vi "Time String to Millisecond.vi"(8 "Error in":errorcluster caption="Error in (no error)", 11 "Parameter":string="1min 30s 20ms") -> (0 "Error out":errorcluster, 2 "Array":string[](array[string]), 3 "sum":i64)   [LabVIEW 2020, in "CSMStand(Lite).lvlib"]
uses:
  CSMStand(Lite).lvlib
  <userlib>/_NEVSTOP/Communicable State Machine(CSM)/addons/API-String-Arugments-Support/API String Arguments Support.lvlib
  <userlib>/_NEVSTOP/Communicable State Machine(CSM)/_Shared/CSM Shared.lvlib
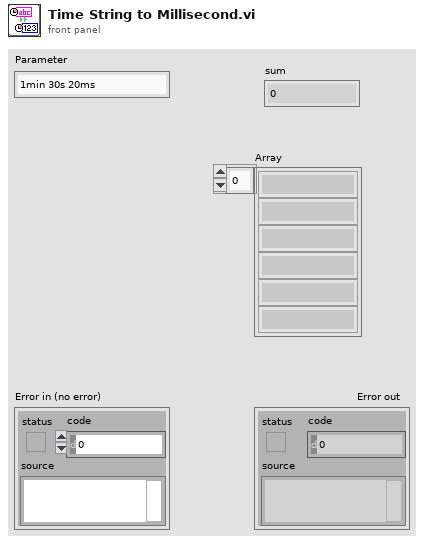
[diagram p1: front panel]
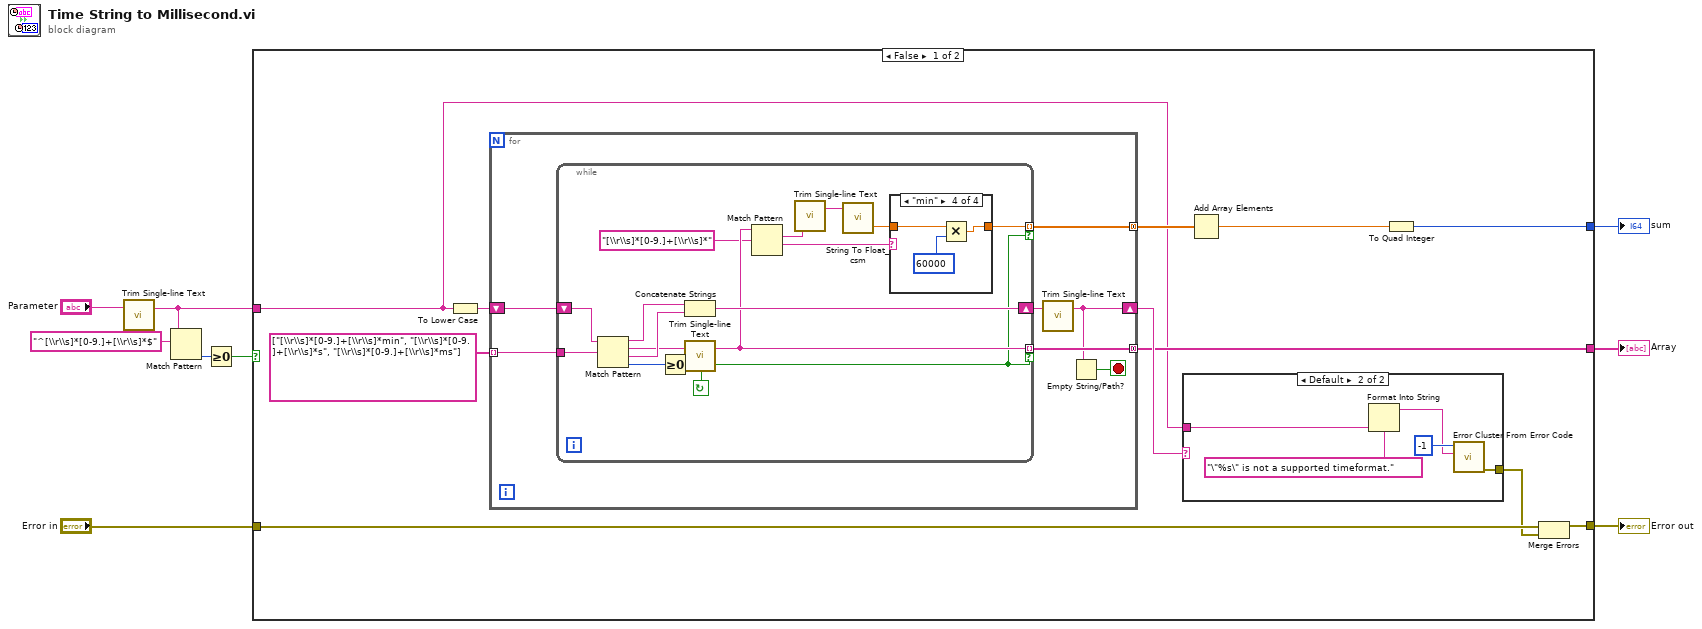
[diagram p0: block diagram]
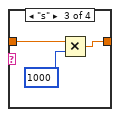
[diagram p5: hidden frame]
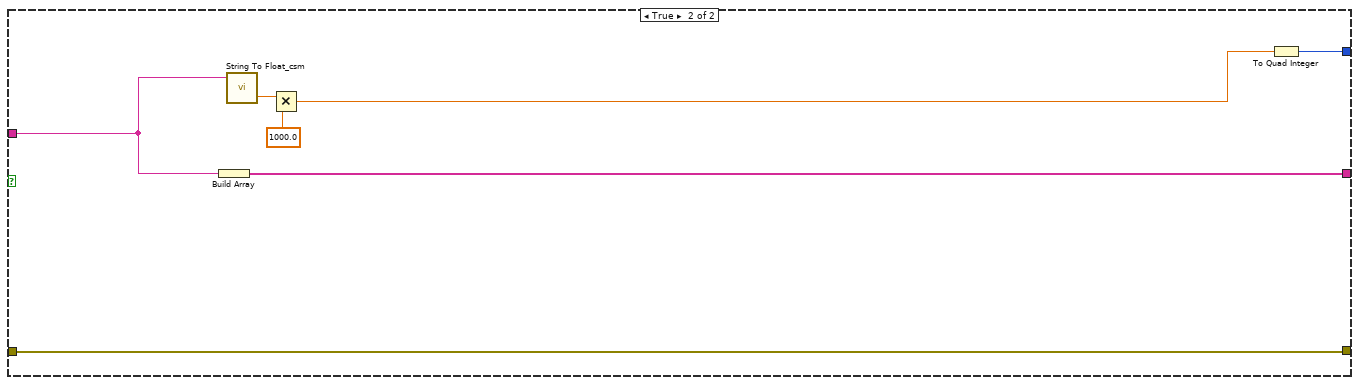
[diagram p6: hidden frame]
diagram:
  n1 = call <userlib>:"Trim Single-line Text.vi"("single-line text"="Parameter") -> ("trimed text"=w1:string)  [unwired: 2 in]
  n2 = Match Pattern(string=w1, regular expression="^[\\r\\s]*[0-9.]+[\\r\\s]*$") -> (offset past match=w3:i32)  [unwired: 1 in, 3 out]
  n3 = Greater Or Equal To 0?(x=w3) -> (x >= 0?=w2:bool)
  n4 = case shown="False" w2 {
    tunnel: "Error in" -> [w18 w61]
    tunnel: [w17 w61] -> w8
    tunnel: [w14 w59] -> w6
    tunnel: [w10 w55] -> w5
    tunnel: w1 -> [w11 w60]
    frame False {
      n5 = To Lower Case(string=w11) -> (all lower case string=w19:string)
      n6 = for {
        shift-right: [w26] -> w16
        shift-left: w19 -> [w32]
        tunnel: string[] ["[\\r\\s]*[0-9.]+[\\r\\s]*min", "[\\r\\s]*[0-9.]+[\\r\\s]*s", "[\\r\\s]*[0-9.]+[\\r\\s]*ms"] ("regular expression") -> [w31] mode=indexing
        tunnel: [w28] -> w14 mode=concatenating
        tunnel: [w27] -> w13 mode=concatenating
        stop <- w30 stop-if-true
        n7 = while {
          shift-right: [w43] -> w29
          shift-left: w32 -> [w44]
          tunnel: w31 -> [w47]
          tunnel: [w40] -> w28 mode=indexing if=w33
          tunnel: [w34] -> w27 mode=indexing if=w33
          stop <- w33 continue-if-true
          n8 = Match Pattern(string=w44, regular expression=w47) -> (before substring=w46:string, match substring=w42:string, after substring=w45:string, offset past match=w41:i32)  [unwired: 1 in]
          n9 = Greater Or Equal To 0?(x=w41) -> (x >= 0?=w33:bool)
          n10 = Concatenate Strings(w46, w45) -> (w43:string)
          n11 = call <userlib>:"Trim Single-line Text.vi"("single-line text"=w42) -> ("trimed text"=w40:string)  [unwired: 2 in]
          n12 = Match Pattern(string=w40, regular expression="[\\r\\s]*[0-9.]+[\\r\\s]*") -> (match substring=w38:string, after substring=w36:string)  [unwired: 1 in, 2 out]
          n13 = call <userlib>:"Trim Single-line Text.vi"("single-line text"=w38) -> ("trimed text"=w37:string)  [unwired: 2 in]
          n14 = call <userlib>:"String To Float_csm.vi"("String"=w37) -> ("Float"=w35:dbl)  [unwired: 3 in, 1 out]
          n15 = case shown="\"min\"" w36 {
            tunnel: [_ w48 w50 w53] -> w34
            tunnel: w35 -> [_ w48 w51 w54]
            frame Default {
            }
            frame "ms" {
            }
            frame "s" {
              n16 = Multiply(x=w51, y=u64 1000) -> (x*y=w50:dbl)
            }
            frame "min" {
              n17 = Multiply(x=w54, y=u64 60000) -> (x*y=w53:dbl)
            }
          }
        }
        n18 = call <userlib>:"Trim Single-line Text.vi"("single-line text"=w29) -> ("trimed text"=w26:string)  [unwired: 2 in]
        n19 = Empty String/Path?(string/path=w26) -> (empty?=w30:bool)
      }
      n20 = case shown="Default" w16 {
        tunnel: [_ w25] -> w15
        tunnel: w11 -> [_ w21]
        frame "" {
        }
        frame Default {
          n21 = Format Into String(format string="\"%s\" is not a supported timeformat." ("error message (\"\")"), w21) -> (resulting string=w22:string)  [unwired: 2 in, 1 out]
          n22 = call <vilib>:"Error Cluster From Error Code.vi"("error message (\"\")"=w22, "error code (0)"=-1) -> ("error out"=w25:errorcluster)  [unwired: 7 in]
        }
      }
      n23 = Add Array Elements(numeric array=w13) -> (sum=w12:dbl)
      n24 = To Quad Integer(1:w12) -> (0:w10:i64)
      n25 = Merge Errors(w18, w15) -> (w17:errorcluster)
    }
    frame True {
      n26 = Build Array(w60) -> (w59:string[])
      n27 = call <userlib>:"String To Float_csm.vi"("String"=w60) -> ("Float"=w58:dbl)  [unwired: 3 in, 1 out]
      n28 = Multiply(x=w58, y=1000.0) -> (x*y=w56:dbl)
      n29 = To Quad Integer(1:w56) -> (0:w55:i64)
    }
  }
  "Array" <- w6
  "Error out" <- w8
  "sum" <- w5
